vi "Command Start Model.vi"(8 "Password":string, 9 "Username":string, 10 "Remote Model Path":string, 11 "Target IP Address":string) -> (0 "error out":errorcluster)   [LabVIEW 2020]
doc: "This VI will send <b>start-model</b> POST message to the Simulation Engine Web Service running on the Linux-RT target specified by <b> Target IP Address</b>. The Simulation Engine Web Service will command the Simulation Engine to run the model specified by <b>Remote Model Path</b>.\nIf your Linux-RT target specifies a"
uses:
  Web Service/Start Model Request Body.ctl
  Web Service/Endpoints.ctl
  <vilib>/httpClient/POSTBuffer.vi
  <vilib>/httpClient/LabVIEWHTTPClient.lvlib
panel:
  out "headers":string
  out "body":string
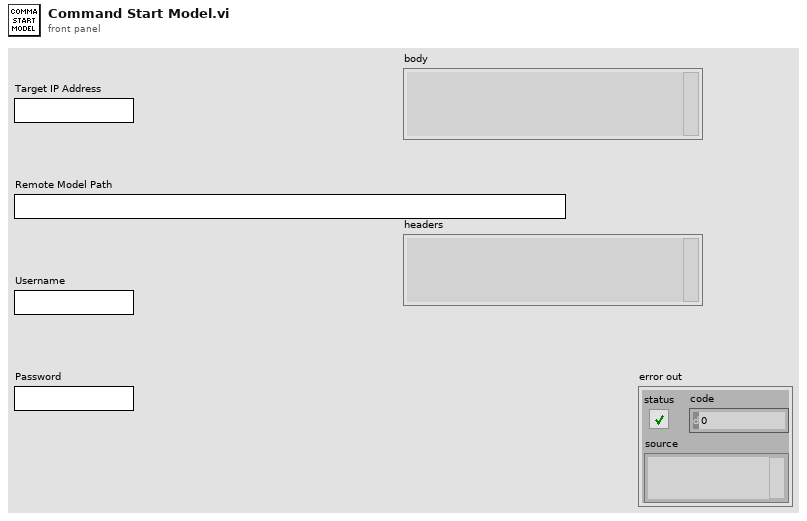
[diagram p1: front panel]
types:
  T1 = typedef "Endpoints.ctl" = string
  T2 = typedef "Start Model Request Body.ctl" = cluster{"ModelPath":string, "SLXRTLibraryPath":string, "ExternalModePort":i32, "SubrateMaxPriority":i32, "SubrateCPUAffinity":i32}
  T3 = typedef "LabVIEWHTTPClient.lvlib/ClientHandle.ctl" = refnum<k1>
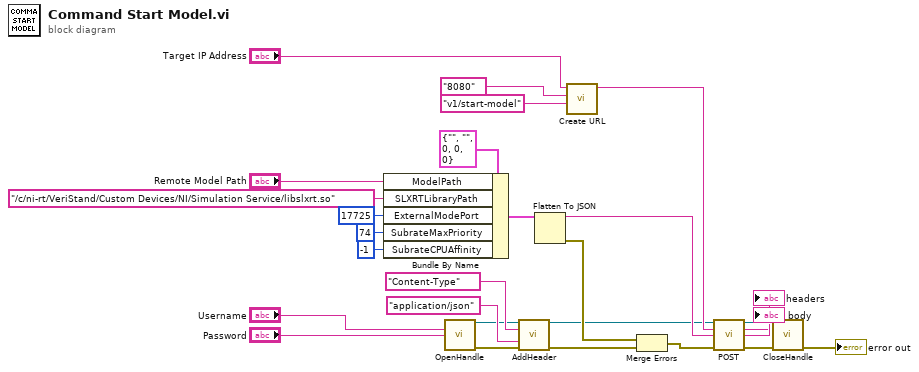
[diagram p0: block diagram]
diagram:
  n1 = Bundle By Name(cluster=T2 {"ModelPath"="", "SLXRTLibraryPath"="", "ExternalModePort"=0, "SubrateMaxPriority"=0, "SubrateCPUAffinity"=0} ("Start Model Request Body"), "ModelPath"="Remote Model Path", "SLXRTLibraryPath"="/c/ni-rt/VeriStand/Custom Devices/NI/Simulation Service/libslxrt.so", "ExternalModePort"=17725, "SubrateMaxPriority"=74, "SubrateCPUAffinity"=-1) -> (w21:T2)
  n2 = call <vilib>:"OpenHandle.vi"("username"="Username", "password"="Password") -> ("client handle out"=w17:T3, "error out"=w14:errorcluster)  [unwired: 12 in]
  n3 = call <vilib>:"AddHeader.vi"("client handle"=w17, "header"="Content-Type", "value"="application/json", "error in (no error)"=w14) -> ("client handle out"=w16:T3, "error out"=w15:errorcluster)  [unwired: 10 in]
  n4 = Flatten To JSON(anything=w21) -> (JSON string=w22:string, 11:w24:errorcluster)  [unwired: 2 in]
  n5 = call "Create URL.vi"("endpoint"=T1 "v1/start-model", "port"="8080", "Target IP Address"="Target IP Address") -> ("URL Out"=w20:string)  [unwired: 8 in]
  n6 = Merge Errors(w24, w15) -> (w23:errorcluster)
  n7 = call-poly <vilib>:"POST.vi"("client handle"=w16, "url"=w20, "buffer"=w22, "error in (no error)"=w23) -> ("client handle out"=w10:T3, "headers"=→"headers":string, "body"=→"body":string, "error out"=w13:errorcluster)  [unwired: 8 in]
  n8 = call <vilib>:"CloseHandle.vi"("client handle"=w10, "error in (no error)"=w13) -> ("error out"=→"error out":errorcluster)  [unwired: 13 in]
